vi "Send-wait-read.vi"(11 "commands":string[](array[string])) -> (1 "All strings":string[](array[string]), 3 "Last string":string)   [LabVIEW 2019]
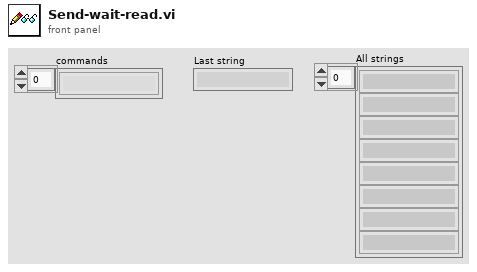
[diagram p1: front panel]
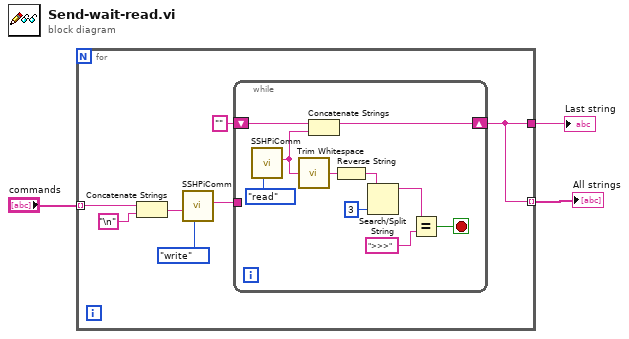
[diagram p0: block diagram]
diagram:
  n1 = for {
    tunnel: "commands" -> [w7] mode=indexing
    tunnel: [w4] -> w2
    tunnel: [w4] -> w1 mode=indexing
    n2 = Concatenate Strings(w7, "\n" ("regular expression")) -> (w6:string)
    n3 = call "SSHPiComm.vi"("Task"=enum16{"init", "read", "write", "close"}."write", "Text to write"=w6) -> ("text read"=w5:string)  [unwired: 8 in, 1 out]
    n4 = while {
      shift-right: [w18] -> w4
      shift-left: "" -> [w19]
      tunnel: w5 -> [_]
      stop <- w11 stop-if-true
      n5 = call "SSHPiComm.vi"("Task"=enum16{"init", "read", "write", "close"}."read") -> ("text read"=w12:string)  [unwired: 9 in, 1 out]
      n6 = call <vilib>:"Trim Whitespace.vi"("string"=w12) -> ("trimmed string"=w17:string)  [unwired: 1 in]
      n7 = Concatenate Strings(w19, w12) -> (w18:string)
      n8 = Reverse String(1:w17) -> (0:w16:string)
      n9 = Search/Split String(string=w16, offset (0)=3) -> (substring before match=w13:string)  [unwired: 1 in, 2 out]
      n10 = Equal?(x=w13, y=">>>") -> (x = y?=w11:bool)
    }
  }
  "Last string" <- w2
  "All strings" <- w1
